vi "CHS_DRIVE_EXECUTE.vi"(6 "Pass_Through_Time":dbl=-1.0 format="%33.4f", 8 "error in (no error)":errorcluster) -> (0 "error out":errorcluster)   [LabVIEW 2019]
uses:
  <vilib>/Rock Robotics/WPI/ThirdParty/JAS_Junk/TrajLib/VI/BoolCmd_Recv_Internal.vi
  <vilib>/Rock Robotics/WPI/ThirdParty/JAS_Junk/TrajLib/VI/numCmd_Recv_Generic.vi
  <vilib>/Rock Robotics/WPI/ThirdParty/JAS_Junk/TrajLib/VI/Util_GetTime_U32.vi
  <vilib>/Rock Robotics/WPI/ThirdParty/JAS_Junk/TrajLib/MathUtil_InputModulus.vi
  <vilib>/Rock Robotics/WPI/ThirdParty/JAS_Junk/TrajLib/VI/BoolCmd_ObtainQueue.vi
  <vilib>/Rock Robotics/WPI/ThirdParty/JAS_Junk/TrajLib/VI/numCmd_ObtainQueue_Generic.vi
  CHS_DRIVE_GLOBALS.vi
  <vilib>/Rock Robotics/SystemInterfaces/Utilities/FPGA_UtilitiesRead LocalTime.vi
  <vilib>/Rock Robotics/WPI/ThirdParty/JAS_Junk/TrajLib/VI/Util_GetTime_U64.vi
  <vilib>/Rock Robotics/WPI/ThirdParty/JAS_Junk/TrajLib/Trajectory_Library.lvlib
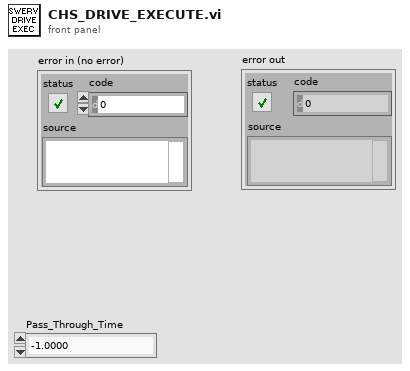
[diagram p1: front panel]
types:
  T1 = typedef "WPI_GyroDevRef.ctl" = cluster{"DevStatus":errorcluster, "Analog Channel":T2, "Gain (VoltsPerDegree/Second)":dbl, "Gyro Type":enum16{"Analog", "XRS450"}, "Handle":i32, "SPI Bus":T3, "Device Found":bool, "Sample Rate":dbl, "Calibrate On Open":bool, "Offset":dbl}
  T2 = typedef "FPGA_AIChannel.ctl" = enum8{"AI 0", "AI 1", "AI 2", "AI 3", "AI MXP 0", "AI MXP 1", "AI MXP 2", "AI MXP 3", "Invalid"}
  T3 = typedef "spi_bus.ctl" = enum16{"SPI On-Board, CS0", "SPI On-Board, CS1", "SPI On-Board, CS2", "SPI On-Board, CS3", "SPI MXP", "Invalid"}
  T4 = typedef "CHS_DRIVE_MODULE_TYPDEF.ctl" = cluster{"SwervDriveMotor":T5, "SwerveSwerveMotor":T5, "SwerveDriveEnc":T10, "SwerveSwerveEnc":T10}
  T5 = typedef "WPI_MotorControlDeviceRef.ctl" = cluster{"DeviceStatus":errorcluster, "Type":T6, "PWM":cluster{"PWM Channel":T7, "DeadBand":T8}, "CAN":cluster{"Device Number":u8, "SetOutput VI Ref":variant, "GetOutput VI Ref":variant, "Enable VI Ref":variant, "Disable VI Ref":variant, "Data":variant}, "Invert":bool, "DIO PWM":cluster{"PWM \"Enable\" Channel":T7, "DIOChannel":T9, "PWM Rate":dbl}}
  T6 = typedef "WPI_MotorControlType.ctl" = enum16{"PWM", "CAN", "DIO PWM"}
  T7 = typedef "FPGA_DIOPWMChannel.ctl" = enum8{"PWM 0", "PWM 1", "PWM 2", "PWM 3", "PWM 4", "PWM 5", "PWM 6", "PWM 7", "PWM 8", "PWM 9", "PWM MXP 0", "PWM MXP 1", "PWM MXP 2", "PWM MXP 3", "PWM MXP 4", "PWM MXP 5", "PWM MXP 6", "PWM MXP 7", "PWM MXP 8", "PWM MXP 9", "Invalid"}
  T8 = typedef "WPI_PWMDeadband.ctl" = cluster{"Name":string, "maxPositivePwm":i32, "minPositivePwm":i32, "centerPwm":i32, "maxNegativePwm":i32, "minNegativePwm":i32, "angularRange":u16}
  T9 = typedef "FPGA_DIOChannel.ctl" = enum8{"DIO 0", "DIO 1", "DIO 2", "DIO 3", "DIO 4", "DIO 5", "DIO 6", "DIO 7", "DIO 8", "DIO 9", "DIO MXP 0", "DIO MXP 1", "DIO MXP 2", "DIO MXP 3", "DIO MXP 4", "DIO MXP 5", "DIO MXP 6", "DIO MXP 7", "DIO MXP 8", "DIO MXP 9", "DIO MXP 10", "DIO MXP 11", "DIO MXP 12", "DIO MXP 13", "DIO MXP 14", "DIO MXP 15", "SPI Port CS1", "SPI Port CS2", "SPI Port CS3", "SPI Port MISO", "SPI Port MOSI", "Invalid"}
  T10 = typedef "WPI_EncoderDevRef.ctl" = cluster{"DevStatus":errorcluster, "EncoderIndex":T11, "CounterIndex":T12, "DistancePerCount":dbl, "Decoding Type":T13}
  T11 = typedef "FPGA_EncoderIdx.ctl" = enum8{"Enc 0", "Enc 1", "Enc 2", "Enc 3", "Enc 4", "Enc 5", "Enc 6", "Enc 7", "Invalid"}
  T12 = typedef "FPGA_CounterCtrSystemIndex.ctl" = enum8{"Ctr 0", "Ctr 1", "Ctr 2", "Ctr 3", "Ctr 4", "Ctr 5", "Ctr 6", "Ctr 7", "Invalid"}
  T13 = typedef "WPI_EncoderType.ctl" = enum16{"1x", "2x", "4x"}
  T14 = typedef "Trajectory_Library.lvlib/SWERVE_DRIVE_MODULE_STATE.ctl" = cluster{"Speed":dbl, "Angle":T15}
  T15 = typedef "Trajectory_Library.lvlib/ROTATION2D.ctl" = cluster{"VALUE":dbl, "COS":dbl, "SIN":dbl}
  T16 = typedef "Trajectory_Library.lvlib/SWERVE_DRIVE_MODULE_POSITION.ctl" = cluster{"Distance":dbl, "Angle":T15, "P":bool}
  T17 = typedef "Trajectory_Library.lvlib/SWERVE_DRIVE_KINEMATICS.ctl" = cluster{"NumModules":i32, "InverseKinematics":T18, "ForwardKinematics":T18, "Modules":T19[], "PrevCoR":T19, "SavedModuleStates":T14[]}
  T18 = typedef "NI_Matrix.lvlib/RealMatrix.ctl" = dbl[][]
  T19 = typedef "Trajectory_Library.lvlib/TRANSLATION2D.ctl" = cluster{"X":dbl, "Y":dbl}
  T20 = typedef "Trajectory_Library.lvlib/CHASSIS_SPEEDS.ctl" = cluster{"vX":dbl, "vY":dbl, "vOmega":dbl}
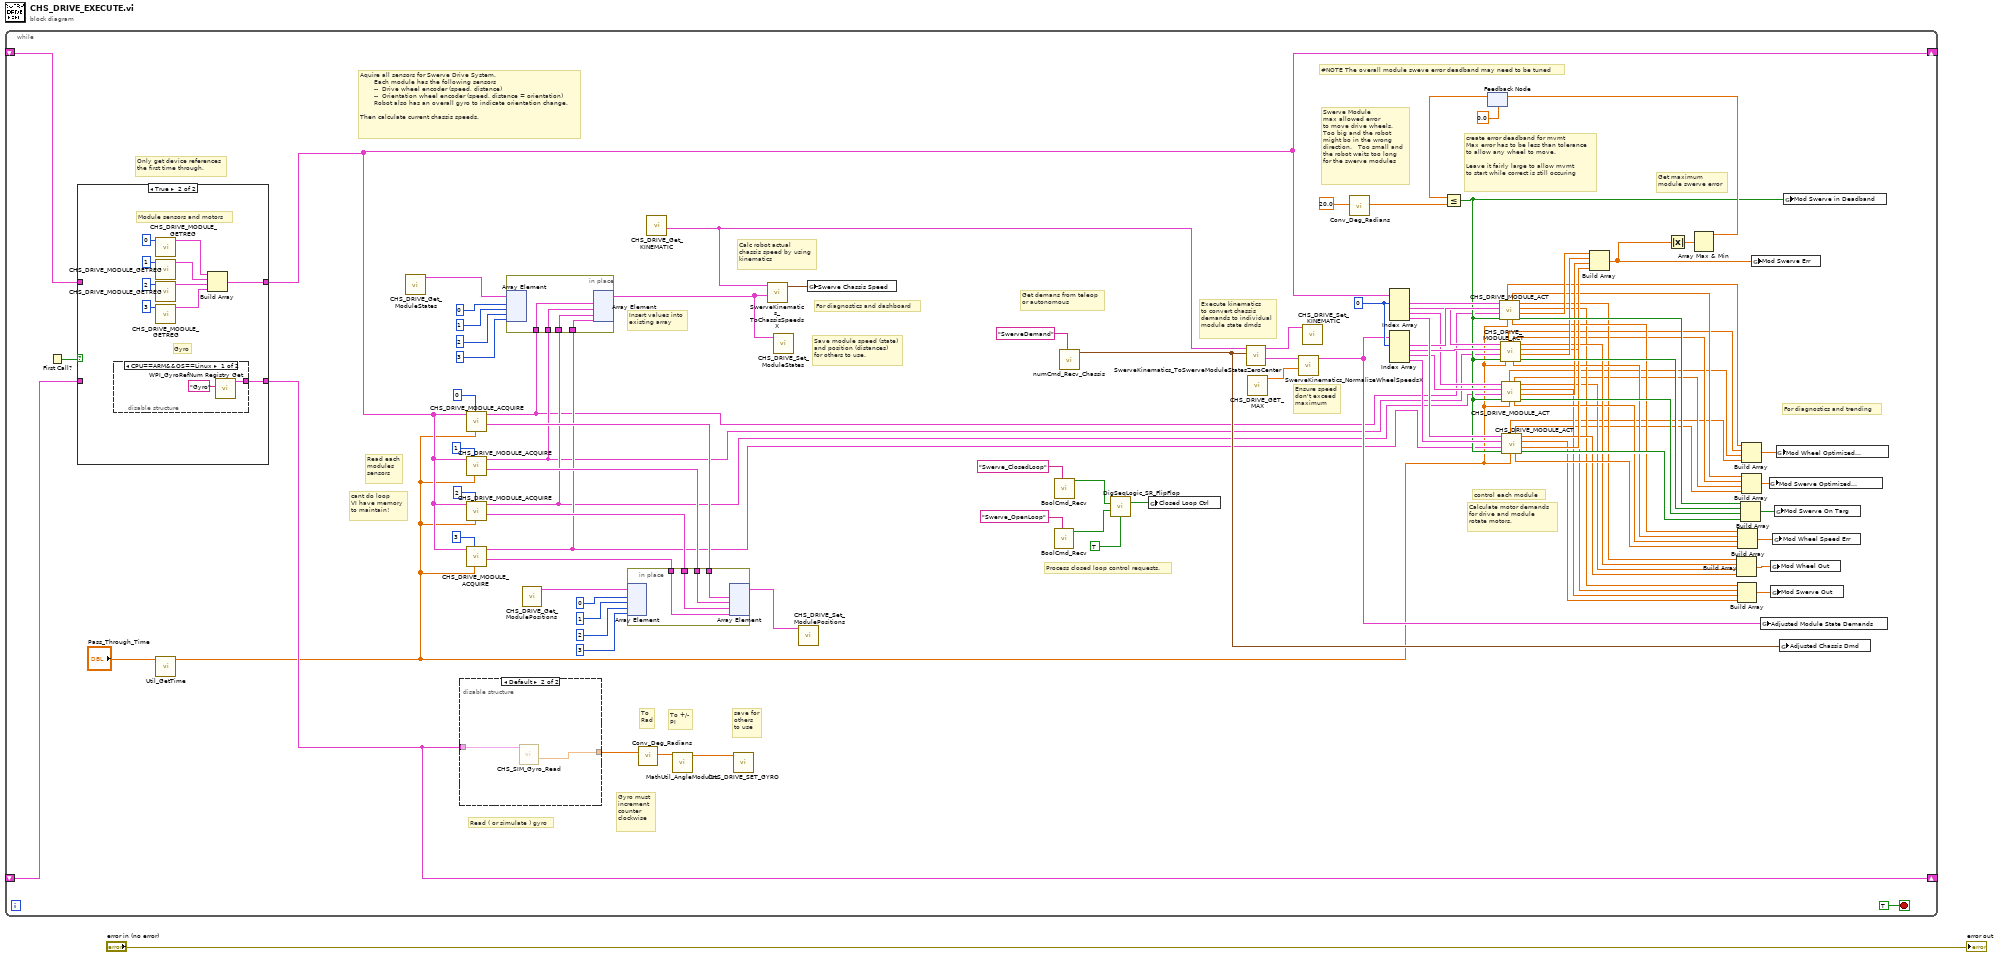
[diagram p0: block diagram]
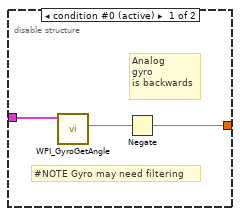
[diagram p4: hidden frame]
diagram:
  n1 = while {
    shift-right: [w25] -> _
    shift-left: _ -> [w26]
    shift-right: [w24] -> _
    shift-left: _ -> [w23]
    stop <- TRUE stop-if-true
    w80 = 0 ("index")
    # "Process closed loop control requests."
    # "Only get device references\nthe first time through."
    # "save for\nothers\nto use"
    # "For diagnostics and trending"
    # "Insert values into\nexisting array"
    # "For diagnostics and dashboard"
    # "Read each\nmodules\nsensors"
    # "Gyro must\nincrement \ncounter\nclockwise"
    # "To +/-\nPI"
    # "To\nRad"
    # "Read ( or simulate ) gyro"
    # "Aquire all sensors for Swerve Drive System.\n       Each module has the following sensors\n       --  Drive wheel encoder (speed, distance)\n       --  Orientation wheel encoder (speed, distance = orientation)\n       Robot also has an overall gyro to indicate orientation change.\n\nThen calculate current chassis speeds."
    # "Calc robot actual\nchassis speed by using\nkinematics"
    # "Save module speed (state)\nand position (distances)\nfor others to use."
    # "cant do loop\nVI have memory\nto maintain!"
    # "Swerve Module\nmax allowed error\nto move drive wheels.\nToo big and the robot\nmight bo in the wrong\ndirection.   Too small and\nthe robot waits too long\nfor the swerve modules"
    # "Ensure speed\ndon't exceed\nmaximum"
    # "Get maximum \nmodule swerve error"
    # "#NOTE The overall module sweve error deadband may need to be tuned"
    # "create error deadband for mvmt\nMax error has to be less than tolerance\nto allow any wheel to move. \n\nLeave it fairly large to allow mvmt\nto start while correct is still occuring"
    # "Calculate motor demands\nfor drive and module \nrotate motors."
    # "Execute kinematics\nto convert chassis \ndemands to individual\nmodule state dmds"
    # "Get demans from teleop\nor autonomous"
    # "control each module"
    n2 = First Call?() -> (First Call?: T/F=w27:bool)
    n3 = case shown="True" w27 {
      tunnel: [w103 w109] -> w25
      tunnel: [w102 w108] -> w24
      tunnel: w26 -> [w103 _]
      tunnel: w23 -> [w102 _]
      frame False {
      }
      frame True {
        # "Module sensors and motors"
        # "Gyro"
        n4 = disable-structure shown="CPU==ARM&&OS==Linux" {
          disable-tunnel: [w114 _] -> w108
          frame condition #0 (active) {
            n5 = call <vilib>:"WPI_GyroRefNum Registry Get.vi"("refnum name"="Gyro") -> ("GyroDevRef"=w114:T1)  [unwired: 9 in, 1 out]
          }
          frame condition #1 {
          }
        }
        n6 = call "CHS_DRIVE_MODULE_GETREG.vi"("Suffix"=0) -> ("Swerve Module TypDef"=w110:T4)  [unwired: 10 in]
        n7 = call "CHS_DRIVE_MODULE_GETREG.vi"("Suffix"=1) -> ("Swerve Module TypDef"=w111:T4)  [unwired: 10 in]
        n8 = call "CHS_DRIVE_MODULE_GETREG.vi"("Suffix"=2) -> ("Swerve Module TypDef"=w112:T4)  [unwired: 10 in]
        n9 = call "CHS_DRIVE_MODULE_GETREG.vi"("Suffix"=3) -> ("Swerve Module TypDef"=w113:T4)  [unwired: 10 in]
        n10 = Build Array(w110, w111, w112, w113) -> (w109:T4[])
      }
    }
    n11 = call <vilib>:"Util_GetTime.vi"("Pass_Through_Time"="Pass_Through_Time") -> ("FPGA_Time_Seconds"=w18:dbl)  [unwired: 8 in, 2 out]
    n12 = call "CHS_DRIVE_Get_ModuleStates.vi"() -> ("Swerve Module States"=w33:T14[])  [unwired: 11 in]
    n13 = disable-structure shown="Default" {
      disable-tunnel: w24 -> [w118 w120]
      disable-tunnel: [w116 w119] -> w36
      frame condition #0 (active) {
        # "Analog\ngyro\nis backwards"
        # "#NOTE Gyro may need filtering"
        n14 = call <vilib>:"WPI_GyroGetAngle.vi"("GyroDevRef"=w118) -> ("Angle"=w117:dbl)  [unwired: 6 in, 4 out]
        n15 = Negate(x=w117) -> (-x=w116:dbl)
      }
      frame condition #1 {
        n16 = call "CHS_SIM_Gyro_Read.vi"("GyroDevRef"=w120) -> ("Gyro_Cont_Deg"=w119:dbl)  [unwired: 10 in]
      }
    }
    n17 = call "CHS_DRIVE_MODULE_ACQUIRE.vi"("Pass_Through_Time"=w18, "Swerve Module Inx"=1, "Swerve Module TypDef"=w25) -> ("SWERVE DRIVE MODULE POSITION"=w43:T16, "Swerve Module State"=w20:T14)  [unwired: 7 in]
    n18 = call "CHS_DRIVE_MODULE_ACQUIRE.vi"("Pass_Through_Time"=w18, "Swerve Module Inx"=3, "Swerve Module TypDef"=w25) -> ("SWERVE DRIVE MODULE POSITION"=w41:T16, "Swerve Module State"=w22:T14)  [unwired: 7 in]
    n19 = call "CHS_DRIVE_MODULE_ACQUIRE.vi"("Pass_Through_Time"=w18, "Swerve Module Inx"=0, "Swerve Module TypDef"=w25) -> ("SWERVE DRIVE MODULE POSITION"=w44:T16, "Swerve Module State"=w8:T14)  [unwired: 7 in]
    n20 = call "CHS_DRIVE_MODULE_ACQUIRE.vi"("Pass_Through_Time"=w18, "Swerve Module Inx"=2, "Swerve Module TypDef"=w25) -> ("SWERVE DRIVE MODULE POSITION"=w42:T16, "Swerve Module State"=w21:T14)  [unwired: 7 in]
    n21 = in-place {
      in-place-border: w8 -> [w124]
      in-place-border: w20 -> [w123]
      in-place-border: w21 -> [w122]
      in-place-border: w22 -> [w121]
      n22 = in-place-array #1(w33, 0, 1, 2, 3) -> ()  [unwired: 4 out]
      n23 = in-place-array #1(w124, w123, w122, w121) -> (w30:T14[])  [unwired: 4 out]
    }
    n24 = call "CHS_DRIVE_Get_ModulePositions.vi"() -> ("Swerve Module Positions"=w32:T16[])  [unwired: 11 in]
    n25 = in-place {
      in-place-border: w44 -> [w128]
      in-place-border: w43 -> [w127]
      in-place-border: w42 -> [w126]
      in-place-border: w41 -> [w125]
      n26 = in-place-array #2(w32, 0, 1, 2, 3) -> ()  [unwired: 4 out]
      n27 = in-place-array #2(w128, w127, w126, w125) -> (w31:T16[])  [unwired: 4 out]
    }
    n28 = call <vilib>:"Conv_Deg_Radians.vi"("Degress"=w36) -> ("Radians"=w54:dbl)  [unwired: 10 in]
    n29 = call "CHS_DRIVE_Get_KINEMATIC.vi"() -> ("out SWERVE_DRIVE_KINEMATICS"=w35:T17)  [unwired: 11 in]
    n30 = call <vilib>:"MathUtil_AngleModulus.vi"("InputAngle"=w54) -> ("ModulsAngle"=w29:dbl)  [unwired: 10 in]
    n31 = call "CHS_DRIVE_SET_GYRO.vi"("Gyro Heading Radians"=w29) -> ()  [unwired: 11 in]
    n32 = call <vilib>:"SwerveKinematics_ToChassisSpeedsX.vi"("WheelStates"=w30, "in SWERVE_DRIVE_KINEMATICS"=w35) -> ("Chassis Speed"=w53:T20)  [unwired: 9 in]
    n33 = call "CHS_DRIVE_Set_ModuleStates.vi"("Swerve Module States"=w30) -> ()  [unwired: 11 in]
    n34 = call "CHS_DRIVE_Set_ModulePositions.vi"("Swerve Module Positions"=w31) -> ()  [unwired: 11 in]
    n35 = global write "CHS_DRIVE_GLOBALS.vi" "Swerve Chassis Speed"(w53) -> ()
    n36 = call <vilib>:"BoolCmd_Recv.vi"("Command Name"="Swerve_OpenLoop") -> ("New Request"=w4:bool)  [unwired: 9 in, 1 out]
    n37 = call <vilib>:"BoolCmd_Recv.vi"("Command Name"="Swerve_ClosedLoop") -> ("New Request"=w5:bool)  [unwired: 9 in, 1 out]
    n38 = call <vilib>:"numCmd_Recv_Chassis.vi"("Command Name"="SwerveDemand") -> ("Chassis Speeds"=w34:T20)  [unwired: 8 in, 2 out]
    n39 = call <vilib>:"DigSeqLogic_SR_FlipFlop.vi"("Set"=w5, "Reset"=w4, "Initial Value"=TRUE) -> ("Output"=w2:bool)  [unwired: 11 in, 1 out]
    n40 = global write "CHS_DRIVE_GLOBALS.vi" "Closed Loop Ctrl"(w2) -> ()
    n41 = call <vilib>:"SwerveKinematics_ToSwerveModuleStatesZeroCenter.vi"("ChassisSpeeds"=w34, "in SWERVE_DRIVE_KINEMATICS"=w35) -> ("ModuleStates"=w67:T14[], "out SWERVE_DRIVE_KINEMATICS"=w57:T17)  [unwired: 8 in]
    n42 = call "CHS_DRIVE_GET_MAX.vi"() -> ("Max Wheel Vel (Meter/Sec)"=w68:dbl)  [unwired: 10 in, 1 out]
    n43 = call <vilib>:"SwerveKinematics_NormalizeWheelSpeedsX.vi"("AttainableMaxSpeed"=w68, "in WheelStates"=w67) -> ("out WheelStates"=w59:T14[])  [unwired: 9 in]
    n44 = call "CHS_DRIVE_Set_KINEMATIC.vi"("SWERVE_DRIVE_KINEMATICS"=w57) -> ()  [unwired: 11 in]
    n45 = call <vilib>:"Conv_Deg_Radians.vi"("Degress"=20.0 ("x")) -> ("Radians"=w56:dbl)  [unwired: 10 in]
    n46 = Index Array(array=w59, index #1=w80) -> (element #1=w72:T14, element #2=w73:T14, element #3=w74:T14, element #4=w84:T14)  [unwired: 3 in]
    n47 = Index Array(array=w25, index #1=w80) -> (element #1=w69:T4, element #2=w70:T4, element #3=w71:T4, element #4=w83:T4)  [unwired: 3 in]
    n48 = feedback #3(0.0) -> (w101:dbl)
    n49 = Less Or Equal?(x=w101, y=w56) -> (x <= y?=w62:bool)
    n50 = call "CHS_DRIVE_MODULE_ACT.vi"("Pass_Through_Time"=w18, "AllSwervePosInDeadband"=w62, "Swerve State"=w8, "Swerve Dmd"=w72, "Swerve Module TypDef"=w69) -> ("SwerveOnTarget"=w94:bool, "SwervePosError"=w89:dbl, "Swerve Motor Dmd"=w77:dbl, "Wheel Motor Dmd"=w75:dbl, "WheelSpeedErr"=w85:dbl, "Optimized Swerve \nDmd Radians"=w19:dbl, "Optimized Speed \nDmd M/S"=w13:dbl)
    n51 = call "CHS_DRIVE_MODULE_ACT.vi"("Pass_Through_Time"=w18, "AllSwervePosInDeadband"=w62, "Swerve State"=w20, "Swerve Dmd"=w73, "Swerve Module TypDef"=w70) -> ("SwerveOnTarget"=w95:bool, "SwervePosError"=w90:dbl, "Swerve Motor Dmd"=w78:dbl, "Wheel Motor Dmd"=w88:dbl, "WheelSpeedErr"=w86:dbl, "Optimized Swerve \nDmd Radians"=w17:dbl, "Optimized Speed \nDmd M/S"=w12:dbl)
    n52 = call "CHS_DRIVE_MODULE_ACT.vi"("Pass_Through_Time"=w18, "AllSwervePosInDeadband"=w62, "Swerve State"=w21, "Swerve Dmd"=w74, "Swerve Module TypDef"=w71) -> ("SwerveOnTarget"=w96:bool, "SwervePosError"=w91:dbl, "Swerve Motor Dmd"=w79:dbl, "Wheel Motor Dmd"=w76:dbl, "WheelSpeedErr"=w87:dbl, "Optimized Swerve \nDmd Radians"=w16:dbl, "Optimized Speed \nDmd M/S"=w11:dbl)
    n53 = call "CHS_DRIVE_MODULE_ACT.vi"("Pass_Through_Time"=w18, "AllSwervePosInDeadband"=w62, "Swerve State"=w22, "Swerve Dmd"=w84, "Swerve Module TypDef"=w83) -> ("SwerveOnTarget"=w97:bool, "SwervePosError"=w92:dbl, "Swerve Motor Dmd"=w82:dbl, "Wheel Motor Dmd"=w81:dbl, "WheelSpeedErr"=w93:dbl, "Optimized Swerve \nDmd Radians"=w15:dbl, "Optimized Speed \nDmd M/S"=w10:dbl)
    n54 = Build Array(w89, w90, w91, w92) -> (w64:dbl[])
    n55 = Absolute Value(x=w64) -> (abs(x)=w98:dbl[])
    n56 = Array Max & Min(array=w98) -> (max value=w99:dbl)  [unwired: 3 out]
    n57 = feedback-in #3(w99) -> ()
    n58 = Build Array(w75, w88, w76, w81) -> (w66:dbl[])
    n59 = Build Array(w77, w78, w79, w82) -> (w65:dbl[])
    n60 = Build Array(w85, w86, w87, w93) -> (w63:dbl[])
    n61 = Build Array(w94, w95, w96, w97) -> (w61:bool[])
    n62 = Build Array(w13, w12, w11, w10) -> (w9:dbl[])
    n63 = Build Array(w19, w17, w16, w15) -> (w14:dbl[])
    n64 = global write "CHS_DRIVE_GLOBALS.vi" "Mod Swerve Err"(w64) -> ()
    n65 = global write "CHS_DRIVE_GLOBALS.vi" "Adjusted Module State Demands"(w59) -> ()
    n66 = global write "CHS_DRIVE_GLOBALS.vi" "Mod Swerve Optimized\nDmd"(w14) -> ()
    n67 = global write "CHS_DRIVE_GLOBALS.vi" "Mod Wheel Out"(w66) -> ()
    n68 = global write "CHS_DRIVE_GLOBALS.vi" "Mod Swerve Out"(w65) -> ()
    n69 = global write "CHS_DRIVE_GLOBALS.vi" "Mod Wheel Speed Err"(w63) -> ()
    n70 = global write "CHS_DRIVE_GLOBALS.vi" "Mod Swerve On Targ"(w61) -> ()
    n71 = global write "CHS_DRIVE_GLOBALS.vi" "Mod Wheel Optimized \nDmd"(w9) -> ()
    n72 = global write "CHS_DRIVE_GLOBALS.vi" "Adjusted Chassis Dmd"(w34) -> ()
    n73 = global write "CHS_DRIVE_GLOBALS.vi" "Mod Swerve in Deadband"(w62) -> ()
  }
  "error out" <- "error in (no error)"
